vi "Determine Clicked Array Element Index.vi"(8 "Error In":errorcluster, 9 "Coords of Click":T1, 11 "Array Refnum":refnum<vi>) -> (0 "Error Out":errorcluster, 1 "Clicked Col":i32, 2 "Clicked Row":i32, 3 "Clicked Index":i32[](array[numeric]), 4 "Horizontal Scroll Clicked?":bool, 5 "Index Display Clicked?":bool, 6 "Vert Scroll Clicked?":bool, 7 "Array Label":string)   [LabVIEW 2021, in "Arrays.lvlib"]
doc: "Determine Clicked Array Element Index.vi\n\n\nDescription:\nThis VI takes the coordinates of click input and determines the index of the array element that the user clicked.\n\nNOTE: Proper operation of the Determine Clicked Array Element Index VI requires that a caption has been created for the array of interest by following the numbered steps below:\n\n(1) Right click on the array of interest and select Visible Items >> Caption\n(The item should be checked)\n\n(2) Right click on the array of interest and select Visible Items >> Caption\n(The item should be un-checked)\n\n(3) Right click on the array of interest and select Visible Items >> Label\n(The item should be checked)\n\n(4) Save the VI\n\nInputs:\nArray Reference - Reference to the array to operate on.\n\nCoords of Click - The screen coordinates of the click within the array. These values are used to determine the index of the array element the user clicked.\n\nOutputs:\nClicked Index - The row and col indices of the item that the user clicked in the array.\n\nClicked Row - The row index of the item that the user clicked in the array.\n\nClicked Col - The column index of the item that the user clicked in the array.\n\nVert Scroll Clicked - Indicates if the vertical scrollbar was clicked.\n\nHorizontal Scroll Clicked - Indicates if the horizontal scrollbar was clicked.\n\nIndex Display Clicked - Indicates if the index display was clicked.\n\nDeveloped By:\nMark.ridgley\nMark.Ridgley_LabVIEW.Developer@comcast.net"
uses:
  Arrays.lvlib
  <vilib>/Utility/miscctls.llb/LVPoint32TypeDef.ctl
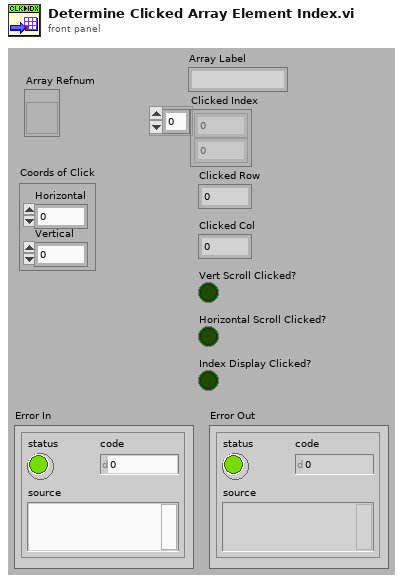
[diagram p1: front panel]
types:
  T1 = typedef "LVPoint32TypeDef.ctl" = cluster{"Horizontal":i32, "Vertical":i32}
  T2 = cluster{"Vertical Scrollbar Visible?":bool, "Vertical Scrollbar Left":i32, "Vertical Scrollbar Right":i32, "Vertical Scrollbar Clicked?":bool, "Horizontal Scrollbar Visible? ":bool, "Horizontal Scrollbar top":i32, "Horizontal Scrollbar Bottom":i32, "Horizontal Scrollbar Clicked?":bool}
  T3 = typedef "LVBoundsTypeDef.ctl" = cluster{"Width":u32, "Height":u32}
  T4 = typedef "LVPositionTypeDef.ctl" = cluster{"Left":i32, "Top":i32}
  T5 = cluster{"Number of Rows":u32, "Number of Columns":u32, "Column Width":u32, "Bounds":T3, "Position":T4, "Array Element.Position":T4, "Index Values":u32[], "Column Left Coordinates":i32[], "Row Top Coordinates":i32[], "Index Display Clicked?":bool, "Element Gap Displayed?":bool}
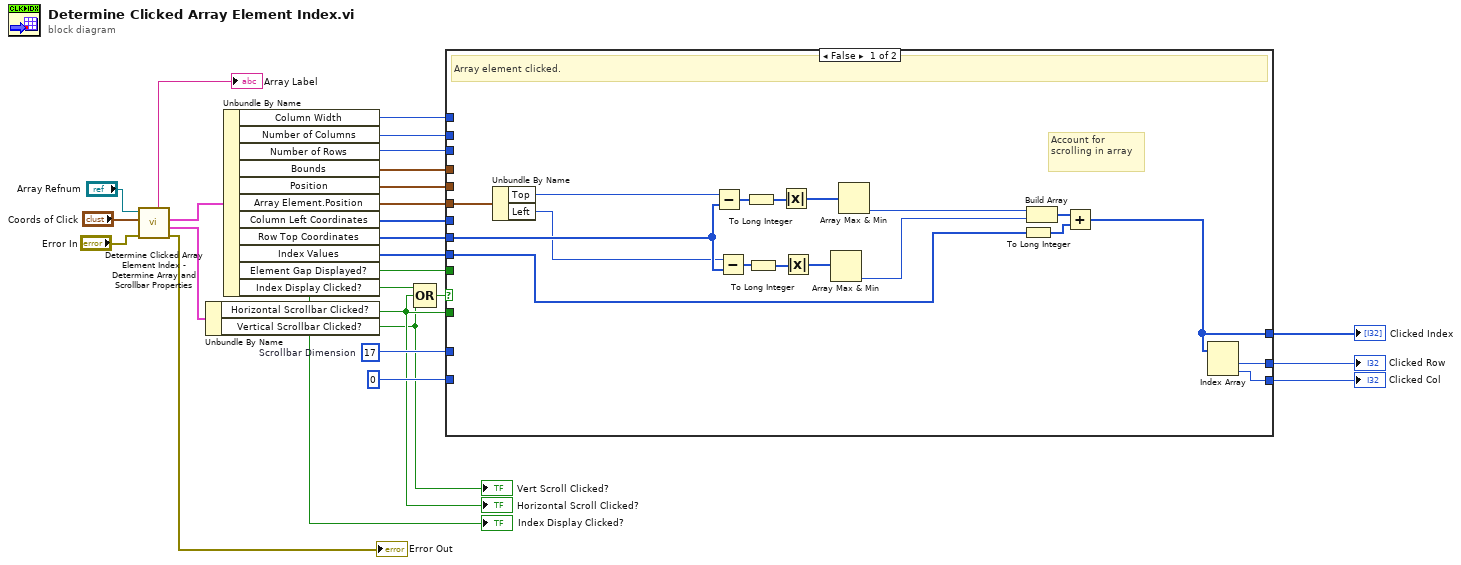
[diagram p0: block diagram]
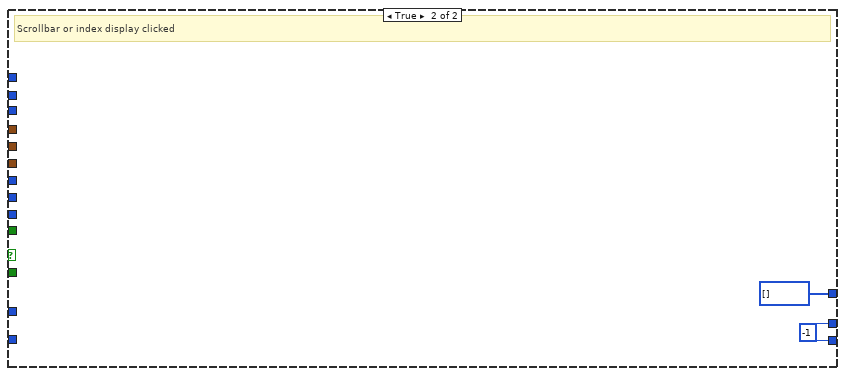
[diagram p2: hidden frame]
diagram:
  w21 = u32 17  # Scrollbar Dimension
  n1 = call "Determine Clicked Array Element Index - Determine Array and Scrollbar Properties.vi"("error in (no error)"="Error In", "Coords of Click"="Coords of Click", "Array Reference"="Array Refnum") -> ("error out"=→"Error Out":errorcluster, "Scrollbar Properties"=w24:T2, "Array Properties"=w25:T5, "Array Label"=→"Array Label":string)  [unwired: 4 in, 1 out]
  n2 = Unbundle By Name(w24) -> ("Horizontal Scrollbar Clicked?"=w17:bool, "Vertical Scrollbar Clicked?"=w13:bool)
  "Horizontal Scroll Clicked?" <- w17
  "Vert Scroll Clicked?" <- w13
  n3 = Unbundle By Name(w25) -> ("Column Width"=w9:u32, "Number of Columns"=w14:u32, "Number of Rows"=w19:u32, "Bounds"=w18:T3, "Position"=w16:T4, "Array Element.Position"=w7:T4, "Column Left Coordinates"=w11:i32[], "Row Top Coordinates"=w12:i32[], "Index Values"=w15:u32[], "Element Gap Displayed?"=w8:bool, "Index Display Clicked?"=w10:bool)
  "Index Display Clicked?" <- w10
  n4 = Compound Arithmetic op=OR(w10, w17, w13) -> (w5:bool)
  n5 = case shown="False" w5 {
    tunnel: w7 -> [w42 _]
    tunnel: [w43 i32[] []] -> w6
    tunnel: w15 -> [w37 _]
    tunnel: w18 -> [_ _]
    tunnel: w16 -> [_ _]
    tunnel: w17 -> [_ _]
    tunnel: w21 -> [_ _]
    tunnel: u32 0 ("Number of Rows") -> [_ _]
    tunnel: w14 -> [_ _]
    tunnel: w19 -> [_ _]
    tunnel: w12 -> [w38 _]
    tunnel: w11 -> [_ _]
    tunnel: w9 -> [_ _]
    tunnel: w8 -> [_ _]
    tunnel: [w28 w45] -> w4
    tunnel: [w27 w45] -> w3
    frame False {
      # "Account for scrolling in array"
      # "Array element clicked."
      n6 = Unbundle By Name(w42) -> ("Top"=w36:i32, "Left"=w32:i32)
      n7 = Subtract(x=w36, y=w38) -> (x-y=w35:i32[])
      n8 = Subtract(x=w32, y=w38) -> (x-y=w30:i32[])
      n9 = To Long Integer(number=w35) -> (32bit integer=w33:i32[])
      n10 = To Long Integer(number=w30) -> (32bit integer=w31:i32[])
      n11 = Absolute Value(x=w33) -> (abs(x)=w34:i32[])
      n12 = Absolute Value(x=w31) -> (abs(x)=w29:i32[])
      n13 = Array Max & Min(array=w29) -> (min index (indices)=w39:i32)  [unwired: 3 out]
      n14 = Array Max & Min(array=w34) -> (min index (indices)=w40:i32)  [unwired: 3 out]
      n15 = To Long Integer(number=w37) -> (32bit integer=w41:i32[])
      n16 = Build Array(w40, w39) -> (w44:i32[])
      n17 = Add(x=w44, y=w41) -> (x+y=w43:i32[])
      n18 = Index Array(array=w43) -> (element #1=w28:i32, element #2=w27:i32)  [unwired: 2 in]
    }
    frame True {
      w45 = -1
      # "Scrollbar or index display clicked"
    }
  }
  "Clicked Index" <- w6
  "Clicked Row" <- w4
  "Clicked Col" <- w3
